vi "Intersection With Configurable Controllers.vi"() -> ()   [LabVIEW 2023]
uses:
  <extravilib>/ChannelInstances/One Element Stream-u16/Read With Abort.vi
  <extravilib>/ChannelInstances/One Element Stream-bool/Instantiate.vi
  <extravilib>/ChannelInstances/One Element Stream-u16/Instantiate.vi
  <extravilib>/ChannelInstances/One Element Stream-u16/EndpointRead.vi
  <extravilib>/ChannelInstances/One Element Stream-u16.lvlib
  <extravilib>/ChannelInstances/One Element Stream-bool.lvlib
panel:
  out "ped":u16(ring)=2
  out "ped":u16(ring)
  out "light":u16(ring)=2
  out "light":u16(ring)
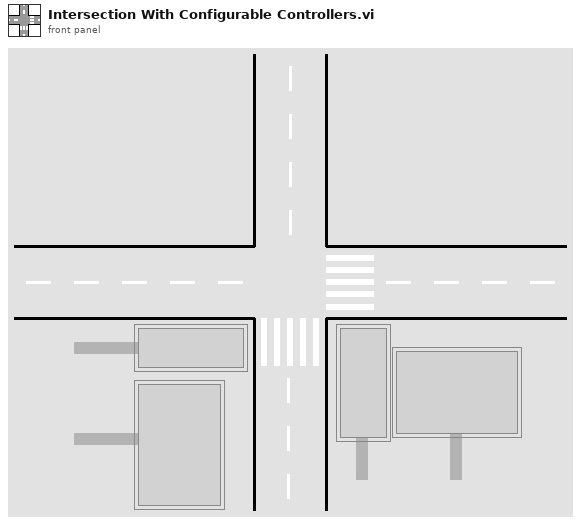
[diagram p1: front panel]
types:
  T1 = typedef "One Element Stream-bool.lvlib/)Channel.ctl" = refnum<queue>
  T2 = typedef "One Element Stream-u16.lvlib/)Channel.ctl" = refnum<queue>
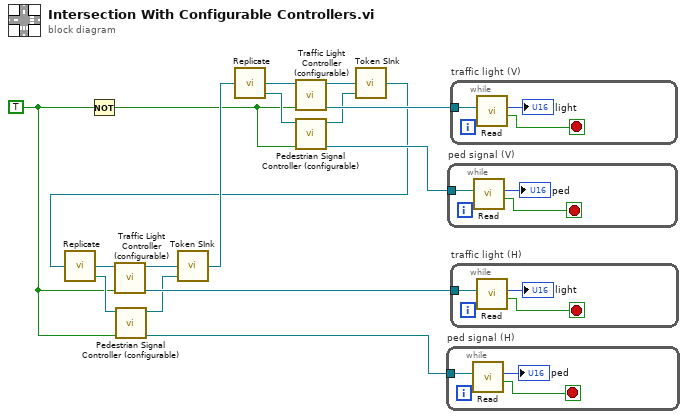
[diagram p0: block diagram]
diagram:
  w2 = TRUE
  n1 = Not(x=w2) -> (.not. x?=w1:bool)
  n2 = call <extravilib>:"Replicate.vi"("one element stream"=w4) -> ("one element stream copy 1"=w11:T1, "one element stream copy 2"=w10:T1)  [unwired: 7 in]
  n3 = call "Traffic Light Controller (configurable).vi"("green"=w2, "peds stopped"=w11) -> ("traffic light"=w16:T2, "cars stopped"=w8:T1)  [unwired: 4 in]
  n4 = call "Pedestrian Signal Controller (configurable).vi"("walk"=w2, "cars stopped"=w10) -> ("ped signal"=w9:T2, "peds stopped"=w6:T1)  [unwired: 8 in]
  n5 = call "Token SInk.vi"("token 1"=w8, "token 2"=w6) -> ("token out"=w7:T1)  [unwired: 7 in]
  n6 = call <extravilib>:"Replicate.vi"("one element stream"=w7) -> ("one element stream copy 1"=w13:T1, "one element stream copy 2"=w12:T1)  [unwired: 7 in]
  n7 = call "Traffic Light Controller (configurable).vi"("green"=w1, "peds stopped"=w13) -> ("traffic light"=w15:T2, "cars stopped"=w5:T1)  [unwired: 4 in]
  n8 = call "Pedestrian Signal Controller (configurable).vi"("walk"=w1, "cars stopped"=w12) -> ("ped signal"=w14:T2, "peds stopped"=w3:T1)  [unwired: 8 in]
  n9 = call "Token SInk.vi"("token 1"=w5, "token 2"=w3) -> ("token out"=w4:T1)  [unwired: 7 in]
  n10 = while "ped signal (H)" {
    tunnel: w9 -> [w19]
    stop <- w18 stop-if-true
    n11 = call <extravilib>:"Read.vi"("channel"=w19) -> ("last element?"=w18:bool, "element"=→"ped":u16)  [unwired: 7 in, 2 out]
  }
  n12 = while "ped signal (V)" {
    tunnel: w14 -> [w22]
    stop <- w21 stop-if-true
    n13 = call <extravilib>:"Read.vi"("channel"=w22) -> ("last element?"=w21:bool, "element"=→"ped":u16)  [unwired: 7 in, 2 out]
  }
  n14 = while "traffic light (V)" {
    tunnel: w15 -> [w25]
    stop <- w24 stop-if-true
    n15 = call <extravilib>:"Read.vi"("channel"=w25) -> ("last element?"=w24:bool, "element"=→"light":u16)  [unwired: 7 in, 2 out]
  }
  n16 = while "traffic light (H)" {
    tunnel: w16 -> [w28]
    stop <- w27 stop-if-true
    n17 = call <extravilib>:"Read.vi"("channel"=w28) -> ("last element?"=w27:bool, "element"=→"light":u16)  [unwired: 7 in, 2 out]
  }
